vi "waveform_to_array.vi"(8 "Waveform Array":waveform(dbl)[](array[waveform])) -> (0 "Array":dbl[][](array[numeric]))   [LabVIEW 2016]
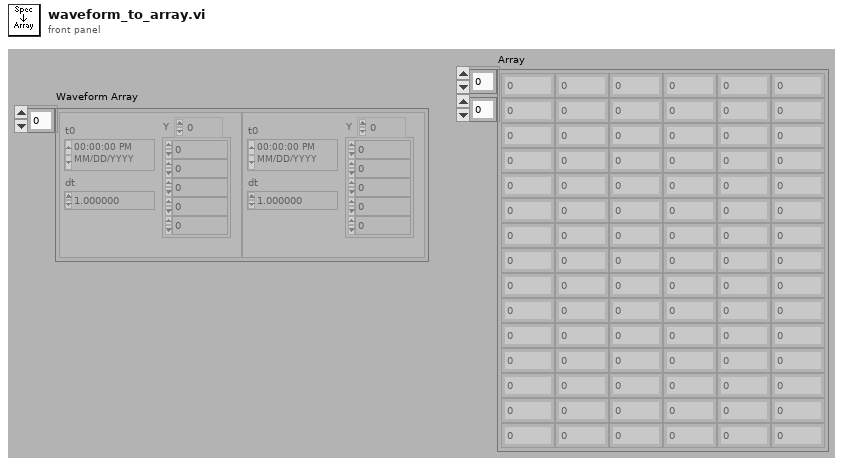
[diagram p1: front panel]
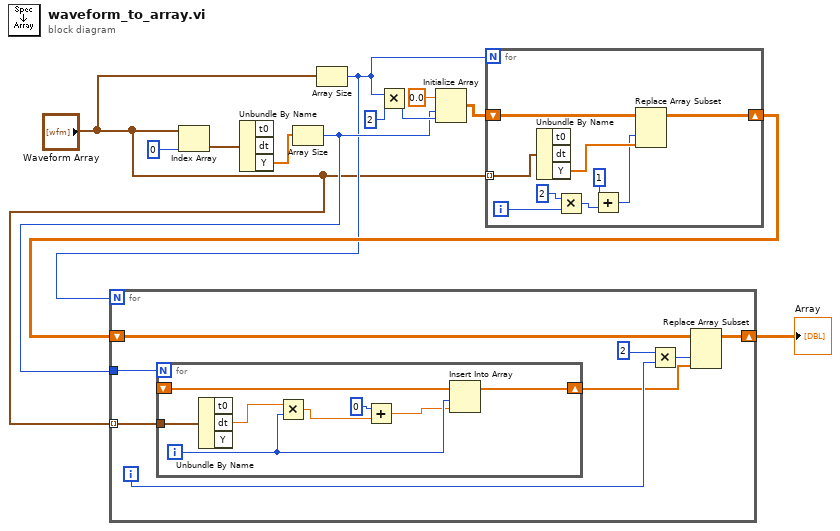
[diagram p0: block diagram]
diagram:
  n1 = Index Array(array="Waveform Array", index=0) -> (element=w4:waveform(dbl))
  n2 = Unbundle By Name(w4) -> ("Y"=w6:dbl[])  [unwired: 2 out]
  n3 = Array Size(array=w6) -> (size(s)=w3:i32)
  n4 = Array Size(array="Waveform Array") -> (size(s)=w2:i32)
  n5 = Multiply(x=w2, y=2) -> (x*y=w7:i32)
  n6 = Initialize Array "Initialize Array"(0.0, w3, w7) -> (w10:dbl[][])
  n7 = for {
    N: w2 -> [_]
    shift-right: [w21] -> w9
    shift-left: w10 -> [w20]
    tunnel: "Waveform Array" -> [w19] mode=indexing
    i -> [w17]
    n8 = Unbundle By Name(w19) -> ("Y"=w18:dbl[])  [unwired: 2 out]
    n9 = Multiply(x=2, y=w17) -> (x*y=w15:i32)
    n10 = Add(x=1, y=w15) -> (x+y=w13:i32)
    n11 = Replace Array Subset "Replace Array Subset"(array=w20, new element=w18, index (col)=w13) -> (w21:dbl[][])  [unwired: 1 in]
  }
  n12 = for {
    N: w2 -> [_]
    shift-right: [w25] -> w5
    shift-left: w9 -> [w29]
    tunnel: w3 -> [w23]
    tunnel: "Waveform Array" -> [w22] mode=indexing
    i -> [w27]
    n13 = for {
      N: w23 -> [_]
      shift-right: [w34] -> w24
      shift-left: _ -> [w33]
      tunnel: w22 -> [w31]
      i -> [w37]
      n14 = Unbundle By Name(w31) -> ("dt"=w30:dbl)  [unwired: 2 out]
      n15 = Multiply(x=w30, y=w37) -> (x*y=w36:dbl)
      n16 = Add(x=0, y=w36) -> (x+y=w35:dbl)
      n17 = Insert Into Array "Insert Into Array"(array=w33, index=w37, new element=w35) -> (w34:dbl[])
    }
    n18 = Multiply(x=2, y=w27) -> (x*y=w26:i32)
    n19 = Replace Array Subset "Replace Array Subset"(array=w29, new element=w24, index (col)=w26) -> (w25:dbl[][])  [unwired: 1 in]
  }
  "Array" <- w5
